vi "Forma Data.vi"(7 "appended array":string[][](array[string]), 8 "error in":errorcluster, 9 "data array":T3 {"data type" items=["Boolean", "SByte", "Byte", "Int16", "UInt16", "Int32", "UInt32", "Int64", "UInt64", "Float", "Double", "String", "DateTime", "ByteString", "Array of Boolean", "Array of SByte", "Array of Byte", "Array of Int16", "Array of UInt16", "Array of Int32", "Array of UInt32", "Array of Int64", "Array of UInt64", "Array of Float", "Array of Double", "Array of String", "Array of DateTime", "Array of ByteString", "Matrix of Boolean", "Matrix of SByte", "Matrix of Byte", "Matrix of Int16", "Matrix of UInt16", "Matrix of Int32", "Matrix of UInt32", "Matrix of Int64", "Matrix of UInt64", "Matrix of Float", "Matrix of Double", "Matrix of String ", "Matrix of DateTime", "Matrix of ByteString"]; "status code" items=["Good"=0, "Good_SubscriptionTransferred"=2949120, "Good_CompletesAsynchronously"=3014656, "Good_Overload"=3080192, "Good_Clamped"=3145728, "Good_LocalOverride"=9830400, "Good_EntryInserted"=10616832, "Good_EntryReplaced"=10682368, "Good_NoData"=10813440, "Good_MoreData"=10878976, "Good_CommunicationEvent"=10944512, "Good_ShutdownEvent"=11010048, "Good_CallAgain"=11075584, "Good_NonCriticalTimeout"=11141120, "Good_ResultsMayBeIncomplete"=12189696, "Good_DataIgnored"=14221312, "Uncertain"=1073741824, "Uncertain_ReferenceOutOfServer"=1080819712, "Uncertain_NoCommunicationLastUsableValue"=1083113472, "Uncertain_LastUsableValue"=1083179008, "Uncertain_SubstituteValue"=1083244544, "Uncertain_InitialValue"=1083310080, "Uncertain_SensorNotAccurate"=1083375616, "Uncertain_EngineeringUnitsExceeded"=1083441152, "Uncertain_SubNormal"=1083506688, "Uncertain_DataSubNormal"=1084489728, "Uncertain_ReferenceNotDeleted"=1086062592, "Uncertain_NotAllNodesAvailable"=1086324736, "Bad"=2147483648, "Bad_UnexpectedError"=2147549184, "Bad_InternalError"=2147614720, "Bad_OutOfMemory"=2147680256, "Bad_ResourceUnavailable"=2147745792, "Bad_CommunicationError"=2147811328, "Bad_EncodingError"=2147876864, "Bad_DecodingError"=2147942400, "Bad_EncodingLimitsExceeded"=2148007936, "Bad_UnknownResponse"=2148073472, "Bad_Timeout"=2148139008, "Bad_ServiceUnsupported"=2148204544, "Bad_Shutdown"=2148270080, "Bad_ServerNotConnected"=2148335616, "Bad_ServerHalted"=2148401152, "Bad_NothingToDo"=2148466688, "Bad_TooManyOperations"=2148532224, "Bad_DataTypeIdUnknown"=2148597760, "Bad_CertificateInvalid"=2148663296, "Bad_SecurityChecksFailed"=2148728832, "Bad_CertificateTimeInvalid"=2148794368, "Bad_CertificateIssuerTimeInvalid"=2148859904, "Bad_CertificateHostNameInvalid"=2148925440, "Bad_CertificateUriInvalid"=2148990976, "Bad_CertificateUseNotAllowed"=2149056512, "Bad_CertificateIssuerUseNotAllowed"=2149122048, "Bad_CertificateUntrusted"=2149187584, "Bad_CertificateRevocationUnknown"=2149253120, "Bad_CertificateIssuerRevocationUnknown"=2149318656, "Bad_CertificateRevoked"=2149384192, "Bad_CertificateIssuerRevoked"=2149449728, "Bad_UserAccessDenied"=2149515264, "Bad_IdentityTokenInvalid"=2149580800, "Bad_IdentityTokenRejected"=2149646336, "Bad_SecureChannelIdInvalid"=2149711872, "Bad_InvalidTimestamp"=2149777408, "Bad_NonceInvalid"=2149842944, "Bad_SessionIdInvalid"=2149908480, "Bad_SessionClosed"=2149974016, "Bad_SessionNotActivated"=2150039552, "Bad_SubscriptionIdInvalid"=2150105088, "Bad_RequestHeaderInvalid"=2150236160, "Bad_TimestampsToReturnInvalid"=2150301696, "Bad_RequestCancelledByClient"=2150367232, "Bad_NoCommunication"=2150694912, "Bad_WaitingForInitialData"=2150760448, "Bad_NodeIdInvalid"=2150825984, "Bad_NodeIdUnknown"=2150891520, "Bad_AttributeIdInvalid"=2150957056, "Bad_IndexRangeInvalid"=2151022592, "Bad_IndexRangeNoData"=2151088128, "Bad_DataEncodingInvalid"=2151153664, "Bad_DataEncodingUnsupported"=2151219200, "Bad_NotReadable"=2151284736, "Bad_NotWritable"=2151350272, "Bad_OutOfRange"=2151415808, "Bad_NotSupported"=2151481344, "Bad_NotFound"=2151546880, "Bad_ObjectDeleted"=2151612416, "Bad_NotImplemented"=2151677952, "Bad_MonitoringModeInvalid"=2151743488, "Bad_MonitoredItemIdInvalid"=2151809024, "Bad_MonitoredItemFilterInvalid"=2151874560, "Bad_MonitoredItemFilterUnsupported"=2151940096, "Bad_FilterNotAllowed"=2152005632, "Bad_StructureMissing"=2152071168, "Bad_EventFilterInvalid"=2152136704, "Bad_ContentFilterInvalid"=2152202240, "Bad_FilterOperandInvalid"=2152267776, "Bad_ContinuationPointInvalid"=2152333312, "Bad_NoContinuationPoints"=2152398848, "Bad_ReferenceTypeIdInvalid"=2152464384, "Bad_BrowseDirectionInvalid"=2152529920, "Bad_NodeNotInView"=2152595456, "Bad_ServerUriInvalid"=2152660992, "Bad_ServerNameMissing"=2152726528, "Bad_DiscoveryUrlMissing"=2152792064, "Bad_SempahoreFileMissing"=2152857600, "Bad_RequestTypeInvalid"=2152923136, "Bad_SecurityModeRejected"=2152988672, "Bad_SecurityPolicyRejected"=2153054208, "Bad_TooManySessions"=2153119744, "Bad_UserSignatureInvalid"=2153185280, "Bad_ApplicationSignatureInvalid"=2153250816, "Bad_NoValidCertificates"=2153316352, "Bad_RequestCancelledByRequest"=2153381888, "Bad_ParentNodeIdInvalid"=2153447424, "Bad_ReferenceNotAllowed"=2153512960, "Bad_NodeIdRejected"=2153578496, "Bad_NodeIdExists"=2153644032, "Bad_NodeClassInvalid"=2153709568, "Bad_BrowseNameInvalid"=2153775104, "Bad_BrowseNameDuplicated"=2153840640, "Bad_NodeAttributesInvalid"=2153906176, "Bad_TypeDefinitionInvalid"=2153971712, "Bad_SourceNodeIdInvalid"=2154037248, "Bad_TargetNodeIdInvalid"=2154102784, "Bad_DuplicateReferenceNotAllowed"=2154168320, "Bad_InvalidSelfReference"=2154233856, "Bad_ReferenceLocalOnly"=2154299392, "Bad_NoDeleteRights"=2154364928, "Bad_ServerIndexInvalid"=2154430464, "Bad_ViewIdUnknown"=2154496000, "Bad_TooManyMatches"=2154627072, "Bad_QueryTooComplex"=2154692608, "Bad_NoMatch"=2154758144, "Bad_MaxAgeInvalid"=2154823680, "Bad_HistoryOperationInvalid"=2154889216, "Bad_HistoryOperationUnsupported"=2154954752, "Bad_WriteNotSupported"=2155020288, "Bad_TypeMismatch"=2155085824, "Bad_MethodInvalid"=2155151360, "Bad_ArgumentsMissing"=2155216896, "Bad_TooManySubscriptions"=2155282432, "Bad_TooManyPublishRequests"=2155347968, "Bad_NoSubscription"=2155413504, "Bad_SequenceNumberUnknown"=2155479040, "Bad_MessageNotAvailable"=2155544576, "Bad_InsufficientClientProfile"=2155610112, "Bad_TcpServerTooBusy"=2155675648, "Bad_TcpMessageTypeInvalid"=2155741184, "Bad_TcpSecureChannelUnknown"=2155806720, "Bad_TcpMessageTooLarge"=2155872256, "Bad_TcpNotEnoughResources"=2155937792, "Bad_TcpInternalError"=2156003328, "Bad_TcpEndpointUrlInvalid"=2156068864, "Bad_RequestInterrupted"=2156134400, "Bad_RequestTimeout"=2156199936, "Bad_SecureChannelClosed"=2156265472, "Bad_SecureChannelTokenUnknown"=2156331008, "Bad_SequenceNumberInvalid"=2156396544, "Bad_ConfigurationError"=2156462080, "Bad_NotConnected"=2156527616, "Bad_DeviceFailure"=2156593152, "Bad_SensorFailure"=2156658688, "Bad_OutOfService"=2156724224, "Bad_DeadbandFilterInvalid"=2156789760, "Bad_RefreshInProgress"=2157379584, "Bad_ConditionAlreadyDisabled"=2157445120, "Bad_ConditionDisabled"=2157510656, "Bad_EventIdUnknown"=2157576192, "Bad_NoData"=2157641728, "Bad_DataLost"=2157772800, "Bad_DataUnavailable"=2157838336, "Bad_EntryExists"=2157903872, "Bad_NoEntryExists"=2157969408, "Bad_TimestampNotSupported"=2158034944, "Bad_InvalidArgument"=2158690304, "Bad_ConnectionRejected"=2158755840, "Bad_Disconnect"=2158821376, "Bad_ConnectionClosed"=2158886912, "Bad_InvalidState"=2158952448, "Bad_EndOfStream"=2159017984, "Bad_NoDataAvailable"=2159083520, "Bad_WaitingForResponse"=2159149056, "Bad_OperationAbandoned"=2159214592, "Bad_ExpectedStreamToBlock"=2159280128, "Bad_WouldBlock"=2159345664, "Bad_SyntaxError"=2159411200, "Bad_MaxConnectionsReached"=2159476736, "Bad_RequestTooLarge"=2159542272, "Bad_ResponseTooLarge"=2159607808, "Bad_EventNotAcknowledgeable"=2159738880, "Bad_InvalidTimestampArgument"=2159869952, "Bad_ProtocolVersionUnsupported"=2159935488, "Bad_StateNotActive"=2160001024, "Bad_FilterOperatorInvalid"=2160132096, "Bad_FilterOperatorUnsupported"=2160197632, "Bad_FilterOperandCountMismatch"=2160263168, "Bad_FilterElementInvalid"=2160328704, "Bad_FilterLiteralInvalid"=2160394240, "Bad_IdentityChangeNotSupported"=2160459776, "Bad_NotTypeDefinition"=2160590848, "Bad_ViewTimestampInvalid"=2160656384, "Bad_ViewParameterMismatch"=2160721920, "Bad_ViewVersionInvalid"=2160787456, "Bad_ConditionAlreadyEnabled"=2160852992, "Bad_DialogNotActive"=2160918528, "Bad_DialogResponseInvalid"=2160984064, "Bad_ConditionBranchAlreadyAcked"=2161049600, "Bad_ConditionBranchAlreadyConfirmed"=2161115136, "Bad_ConditionAlreadyShelved"=2161180672, "Bad_ConditionNotShelved"=2161246208, "Bad_ShelvingTimeOutOfRange"=2161311744, "Bad_AggregateListMismatch"=2161377280, "Bad_AggregateNotSupported"=2161442816, "Bad_AggregateInvalidInputs"=2161508352, "Bad_BoundNotFound"=2161573888, "Bad_BoundNotSupported"=2161639424, "Bad_AggregateConfigurationRejected"=2161770496, "Bad_TooManyMonitoredItems"=2161836032]}, 10 "type":enum16{"Insert", "Replace", "Append"}(ring), 11 "Multicolumn Listbox":refnum<vi>) -> (0 "error out":errorcluster, 1 "Alarm Summary Data":string[][](array[string]), 2 "Alarm Summary Headers":string[](array[string]), 3 "dup Multicolumn Listbox":refnum<vi>)   [LabVIEW 2019]
uses:
  Alarm Description Item.ctl
  Control 1.ctl
  <vilib>/OPCUA/controls/Subscription Data Change.ctl
  <vilib>/OPCUA/controls/NodeId.ctl
  <vilib>/OPCUA/controls/Data Type.ctl
  <vilib>/OPCUA/controls/OPC UA StatusCode.ctl
panel:
  out "data type":T1=1 items=["Boolean", "SByte", "Byte", "Int16", "UInt16", "Int32", "UInt32", "Int64", "UInt64", "Float", "Double", "String", "DateTime", "ByteString", "Array of Boolean", "Array of SByte", "Array of Byte", "Array of Int16", "Array of UInt16", "Array of Int32", "Array of UInt32", "Array of Int64", "Array of UInt64", "Array of Float", "Array of Double", "Array of String", "Array of DateTime", "Array of ByteString", "Matrix of Boolean", "Matrix of SByte", "Matrix of Byte", "Matrix of Int16", "Matrix of UInt16", "Matrix of Int32", "Matrix of UInt32", "Matrix of Int64", "Matrix of UInt64", "Matrix of Float", "Matrix of Double", "Matrix of String ", "Matrix of DateTime", "Matrix of ByteString"]
  out "Status Code":T2 items=["Good"=0, "Good_SubscriptionTransferred"=2949120, "Good_CompletesAsynchronously"=3014656, "Good_Overload"=3080192, "Good_Clamped"=3145728, "Good_LocalOverride"=9830400, "Good_EntryInserted"=10616832, "Good_EntryReplaced"=10682368, "Good_NoData"=10813440, "Good_MoreData"=10878976, "Good_CommunicationEvent"=10944512, "Good_ShutdownEvent"=11010048, "Good_CallAgain"=11075584, "Good_NonCriticalTimeout"=11141120, "Good_ResultsMayBeIncomplete"=12189696, "Good_DataIgnored"=14221312, "Uncertain"=1073741824, "Uncertain_ReferenceOutOfServer"=1080819712, "Uncertain_NoCommunicationLastUsableValue"=1083113472, "Uncertain_LastUsableValue"=1083179008, "Uncertain_SubstituteValue"=1083244544, "Uncertain_InitialValue"=1083310080, "Uncertain_SensorNotAccurate"=1083375616, "Uncertain_EngineeringUnitsExceeded"=1083441152, "Uncertain_SubNormal"=1083506688, "Uncertain_DataSubNormal"=1084489728, "Uncertain_ReferenceNotDeleted"=1086062592, "Uncertain_NotAllNodesAvailable"=1086324736, "Bad"=2147483648, "Bad_UnexpectedError"=2147549184, "Bad_InternalError"=2147614720, "Bad_OutOfMemory"=2147680256, "Bad_ResourceUnavailable"=2147745792, "Bad_CommunicationError"=2147811328, "Bad_EncodingError"=2147876864, "Bad_DecodingError"=2147942400, "Bad_EncodingLimitsExceeded"=2148007936, "Bad_UnknownResponse"=2148073472, "Bad_Timeout"=2148139008, "Bad_ServiceUnsupported"=2148204544, "Bad_Shutdown"=2148270080, "Bad_ServerNotConnected"=2148335616, "Bad_ServerHalted"=2148401152, "Bad_NothingToDo"=2148466688, "Bad_TooManyOperations"=2148532224, "Bad_DataTypeIdUnknown"=2148597760, "Bad_CertificateInvalid"=2148663296, "Bad_SecurityChecksFailed"=2148728832, "Bad_CertificateTimeInvalid"=2148794368, "Bad_CertificateIssuerTimeInvalid"=2148859904, "Bad_CertificateHostNameInvalid"=2148925440, "Bad_CertificateUriInvalid"=2148990976, "Bad_CertificateUseNotAllowed"=2149056512, "Bad_CertificateIssuerUseNotAllowed"=2149122048, "Bad_CertificateUntrusted"=2149187584, "Bad_CertificateRevocationUnknown"=2149253120, "Bad_CertificateIssuerRevocationUnknown"=2149318656, "Bad_CertificateRevoked"=2149384192, "Bad_CertificateIssuerRevoked"=2149449728, "Bad_UserAccessDenied"=2149515264, "Bad_IdentityTokenInvalid"=2149580800, "Bad_IdentityTokenRejected"=2149646336, "Bad_SecureChannelIdInvalid"=2149711872, "Bad_InvalidTimestamp"=2149777408, "Bad_NonceInvalid"=2149842944, "Bad_SessionIdInvalid"=2149908480, "Bad_SessionClosed"=2149974016, "Bad_SessionNotActivated"=2150039552, "Bad_SubscriptionIdInvalid"=2150105088, "Bad_RequestHeaderInvalid"=2150236160, "Bad_TimestampsToReturnInvalid"=2150301696, "Bad_RequestCancelledByClient"=2150367232, "Bad_NoCommunication"=2150694912, "Bad_WaitingForInitialData"=2150760448, "Bad_NodeIdInvalid"=2150825984, "Bad_NodeIdUnknown"=2150891520, "Bad_AttributeIdInvalid"=2150957056, "Bad_IndexRangeInvalid"=2151022592, "Bad_IndexRangeNoData"=2151088128, "Bad_DataEncodingInvalid"=2151153664, "Bad_DataEncodingUnsupported"=2151219200, "Bad_NotReadable"=2151284736, "Bad_NotWritable"=2151350272, "Bad_OutOfRange"=2151415808, "Bad_NotSupported"=2151481344, "Bad_NotFound"=2151546880, "Bad_ObjectDeleted"=2151612416, "Bad_NotImplemented"=2151677952, "Bad_MonitoringModeInvalid"=2151743488, "Bad_MonitoredItemIdInvalid"=2151809024, "Bad_MonitoredItemFilterInvalid"=2151874560, "Bad_MonitoredItemFilterUnsupported"=2151940096, "Bad_FilterNotAllowed"=2152005632, "Bad_StructureMissing"=2152071168, "Bad_EventFilterInvalid"=2152136704, "Bad_ContentFilterInvalid"=2152202240, "Bad_FilterOperandInvalid"=2152267776, "Bad_ContinuationPointInvalid"=2152333312, "Bad_NoContinuationPoints"=2152398848, "Bad_ReferenceTypeIdInvalid"=2152464384, "Bad_BrowseDirectionInvalid"=2152529920, "Bad_NodeNotInView"=2152595456, "Bad_ServerUriInvalid"=2152660992, "Bad_ServerNameMissing"=2152726528, "Bad_DiscoveryUrlMissing"=2152792064, "Bad_SempahoreFileMissing"=2152857600, "Bad_RequestTypeInvalid"=2152923136, "Bad_SecurityModeRejected"=2152988672, "Bad_SecurityPolicyRejected"=2153054208, "Bad_TooManySessions"=2153119744, "Bad_UserSignatureInvalid"=2153185280, "Bad_ApplicationSignatureInvalid"=2153250816, "Bad_NoValidCertificates"=2153316352, "Bad_RequestCancelledByRequest"=2153381888, "Bad_ParentNodeIdInvalid"=2153447424, "Bad_ReferenceNotAllowed"=2153512960, "Bad_NodeIdRejected"=2153578496, "Bad_NodeIdExists"=2153644032, "Bad_NodeClassInvalid"=2153709568, "Bad_BrowseNameInvalid"=2153775104, "Bad_BrowseNameDuplicated"=2153840640, "Bad_NodeAttributesInvalid"=2153906176, "Bad_TypeDefinitionInvalid"=2153971712, "Bad_SourceNodeIdInvalid"=2154037248, "Bad_TargetNodeIdInvalid"=2154102784, "Bad_DuplicateReferenceNotAllowed"=2154168320, "Bad_InvalidSelfReference"=2154233856, "Bad_ReferenceLocalOnly"=2154299392, "Bad_NoDeleteRights"=2154364928, "Bad_ServerIndexInvalid"=2154430464, "Bad_ViewIdUnknown"=2154496000, "Bad_TooManyMatches"=2154627072, "Bad_QueryTooComplex"=2154692608, "Bad_NoMatch"=2154758144, "Bad_MaxAgeInvalid"=2154823680, "Bad_HistoryOperationInvalid"=2154889216, "Bad_HistoryOperationUnsupported"=2154954752, "Bad_WriteNotSupported"=2155020288, "Bad_TypeMismatch"=2155085824, "Bad_MethodInvalid"=2155151360, "Bad_ArgumentsMissing"=2155216896, "Bad_TooManySubscriptions"=2155282432, "Bad_TooManyPublishRequests"=2155347968, "Bad_NoSubscription"=2155413504, "Bad_SequenceNumberUnknown"=2155479040, "Bad_MessageNotAvailable"=2155544576, "Bad_InsufficientClientProfile"=2155610112, "Bad_TcpServerTooBusy"=2155675648, "Bad_TcpMessageTypeInvalid"=2155741184, "Bad_TcpSecureChannelUnknown"=2155806720, "Bad_TcpMessageTooLarge"=2155872256, "Bad_TcpNotEnoughResources"=2155937792, "Bad_TcpInternalError"=2156003328, "Bad_TcpEndpointUrlInvalid"=2156068864, "Bad_RequestInterrupted"=2156134400, "Bad_RequestTimeout"=2156199936, "Bad_SecureChannelClosed"=2156265472, "Bad_SecureChannelTokenUnknown"=2156331008, "Bad_SequenceNumberInvalid"=2156396544, "Bad_ConfigurationError"=2156462080, "Bad_NotConnected"=2156527616, "Bad_DeviceFailure"=2156593152, "Bad_SensorFailure"=2156658688, "Bad_OutOfService"=2156724224, "Bad_DeadbandFilterInvalid"=2156789760, "Bad_RefreshInProgress"=2157379584, "Bad_ConditionAlreadyDisabled"=2157445120, "Bad_ConditionDisabled"=2157510656, "Bad_EventIdUnknown"=2157576192, "Bad_NoData"=2157641728, "Bad_DataLost"=2157772800, "Bad_DataUnavailable"=2157838336, "Bad_EntryExists"=2157903872, "Bad_NoEntryExists"=2157969408, "Bad_TimestampNotSupported"=2158034944, "Bad_InvalidArgument"=2158690304, "Bad_ConnectionRejected"=2158755840, "Bad_Disconnect"=2158821376, "Bad_ConnectionClosed"=2158886912, "Bad_InvalidState"=2158952448, "Bad_EndOfStream"=2159017984, "Bad_NoDataAvailable"=2159083520, "Bad_WaitingForResponse"=2159149056, "Bad_OperationAbandoned"=2159214592, "Bad_ExpectedStreamToBlock"=2159280128, "Bad_WouldBlock"=2159345664, "Bad_SyntaxError"=2159411200, "Bad_MaxConnectionsReached"=2159476736, "Bad_RequestTooLarge"=2159542272, "Bad_ResponseTooLarge"=2159607808, "Bad_EventNotAcknowledgeable"=2159738880, "Bad_InvalidTimestampArgument"=2159869952, "Bad_ProtocolVersionUnsupported"=2159935488, "Bad_StateNotActive"=2160001024, "Bad_FilterOperatorInvalid"=2160132096, "Bad_FilterOperatorUnsupported"=2160197632, "Bad_FilterOperandCountMismatch"=2160263168, "Bad_FilterElementInvalid"=2160328704, "Bad_FilterLiteralInvalid"=2160394240, "Bad_IdentityChangeNotSupported"=2160459776, "Bad_NotTypeDefinition"=2160590848, "Bad_ViewTimestampInvalid"=2160656384, "Bad_ViewParameterMismatch"=2160721920, "Bad_ViewVersionInvalid"=2160787456, "Bad_ConditionAlreadyEnabled"=2160852992, "Bad_DialogNotActive"=2160918528, "Bad_DialogResponseInvalid"=2160984064, "Bad_ConditionBranchAlreadyAcked"=2161049600, "Bad_ConditionBranchAlreadyConfirmed"=2161115136, "Bad_ConditionAlreadyShelved"=2161180672, "Bad_ConditionNotShelved"=2161246208, "Bad_ShelvingTimeOutOfRange"=2161311744, "Bad_AggregateListMismatch"=2161377280, "Bad_AggregateNotSupported"=2161442816, "Bad_AggregateInvalidInputs"=2161508352, "Bad_BoundNotFound"=2161573888, "Bad_BoundNotSupported"=2161639424, "Bad_AggregateConfigurationRejected"=2161770496, "Bad_TooManyMonitoredItems"=2161836032]
  in  "alarm display format":T6[](array[typedef])=[enum."Type", enum."Name", enum."Value", enum."time", enum."status code", enum."data type", enum."node ID", enum."Color"]
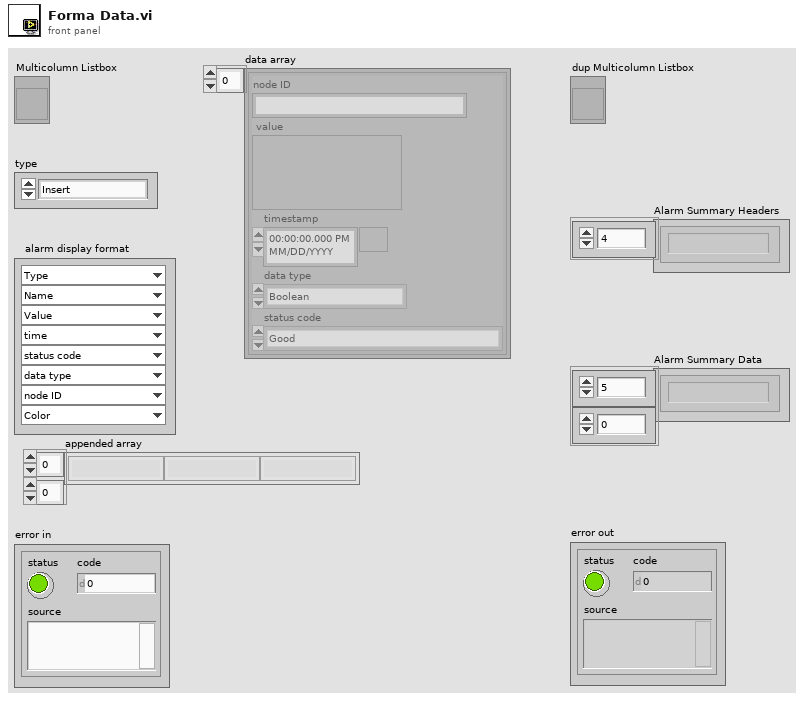
[diagram p1: front panel]
types:
  T1 = typedef "Data Type.ctl" = u16
  T2 = typedef "OPC UA StatusCode.ctl" = u32
  T3 = typedef "Control 1.ctl" = T4[]
  T4 = typedef "Subscription Data Change.ctl" = cluster{"node ID":T5, " value":variant, "timestamp":timestamp, "data type":T1, "status code":T2}
  T5 = typedef "NodeId.ctl" = string
  T6 = typedef "Alarm Description Item.ctl" = enum16{"Type", "Name", "node ID", "Value", "time", "data type", "status code", "Color"}
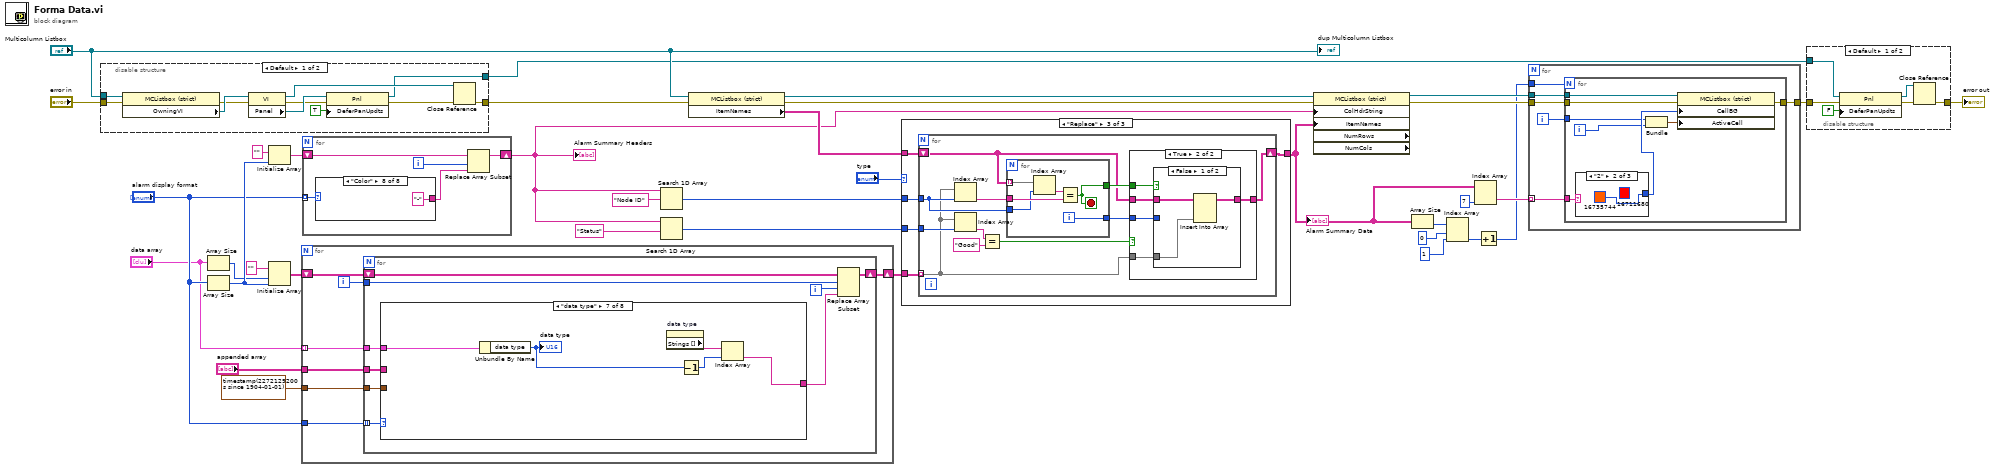
[diagram p0: block diagram]
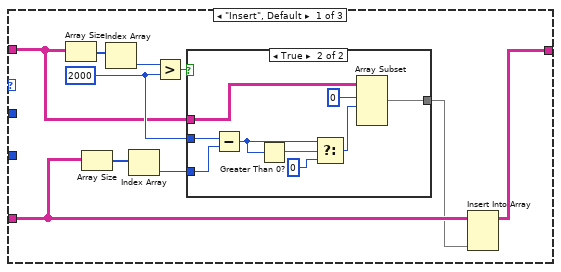
[diagram p4: hidden frame]
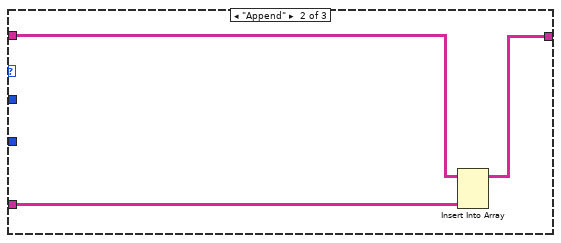
[diagram p6: hidden frame]
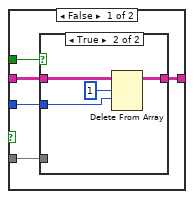
[diagram p7: hidden frame]
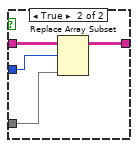
[diagram p9: hidden frame]
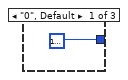
[diagram p10: hidden frame]
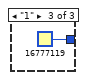
[diagram p11: hidden frame]
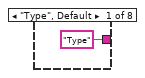
[diagram p12: hidden frame]
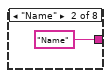
[diagram p13: hidden frame]
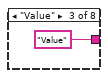
[diagram p14: hidden frame]
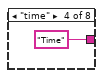
[diagram p15: hidden frame]
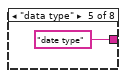
[diagram p16: hidden frame]
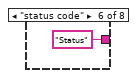
[diagram p17: hidden frame]
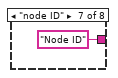
[diagram p18: hidden frame]
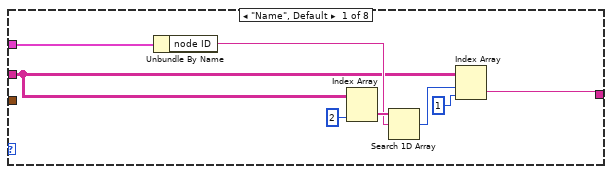
[diagram p19: hidden frame]
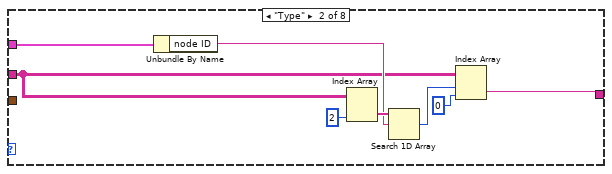
[diagram p20: hidden frame]
diagram:
  n1 = disable-structure shown="Default" {
    disable-tunnel: "error in" -> [w40 w48]
    disable-tunnel: "Multicolumn Listbox" -> [w39 _]
    disable-tunnel: [w38 w48] -> w14
    disable-tunnel: [w37 _] -> w11
    frame condition #0 (active) {
      n2 = property class="MCListbox (strict)"(reference=w39, error in=w40) -> (error out=w46:errorcluster, "OwningVI"=w47:refnum<vi>)  [unwired: 1 out]
      n3 = property class="VI"(reference=w47, error in=w46) -> (reference out=w42:refnum<vi>, error out=w44:errorcluster, "Panel"=w45:refnum<vi>)
      n4 = property class="Pnl"(reference=w45, error in=w44, "DeferPanUpdts"=TRUE ("Defer Panel Updates")) -> (reference out=w37:refnum<vi>, error out=w41:errorcluster)
      n5 = Close Reference(reference=w42, error in (no error)=w41) -> (error out=w38:errorcluster)
    }
    frame condition #1 {
    }
  }
  n6 = Array Size(array="data array") -> (size(s)=w31:i32)
  n7 = Array Size(array="alarm display format") -> (size(s)=w35:i32)
  n8 = Initialize Array("" ("element"), w35) -> (w36:string[])
  n9 = Initialize Array("" ("alarm URL"), w31, w35) -> (w33:string[][])
  n10 = for {
    tunnel: "data array" -> [w50] mode=indexing
    tunnel: "alarm display format" -> [w55]
    shift-right: [w53] -> w21
    shift-left: w33 -> [w54]
    tunnel: timestamp(2272129200 s since 1904-01-01) ("ack time") -> [w51]
    tunnel: "appended array" -> [w49]
    i -> [w52]
    n11 = for {
      tunnel: w55 -> [w64] mode=indexing
      tunnel: w50 -> [w57]
      tunnel: w52 -> [w61]
      shift-right: [w62] -> w53
      shift-left: w54 -> [w63]
      tunnel: w51 -> [w58]
      tunnel: w49 -> [w56]
      i -> [w60]
      n12 = case shown="\"data type\"" w64 {
        tunnel: w57 -> [w72 w80 w92 w100 w107 w112 w121 w125]
        tunnel: [w66 w73 w81 w99 w102 w111 w119 w122] -> w59
        tunnel: w58 -> [_ _ _ _ _ w109 _ _]
        tunnel: w56 -> [w65 w74 w86 _ _ _ _ _]
        frame "Name", Default {
          n13 = Unbundle By Name(w72) -> ("node ID"=w69:T5)
          n14 = Index Array(array=w65, index (col)=2 ("disabled index (col)")) -> (element=w70:string[])  [unwired: 1 in]
          n15 = Search 1D Array(1D array=w70, element=w69) -> (index of element=w67:i32)  [unwired: 1 in]
          n16 = Index Array(array=w65, index (row)=w67, index (col)=1 ("disabled index (col)")) -> (element=w66:string)
        }
        frame "Type" {
          n17 = Unbundle By Name(w80) -> ("node ID"=w77:T5)
          n18 = Index Array(array=w74, index (col)=2 ("disabled index (col)")) -> (element=w78:string[])  [unwired: 1 in]
          n19 = Search 1D Array(1D array=w78, element=w77) -> (index of element=w75:i32)  [unwired: 1 in]
          n20 = Index Array(array=w74, index (row)=w75, index (col)=0 ("disabled index (col)")) -> (element=w73:string)
        }
        frame "Color" {
          n21 = Unbundle By Name(w92) -> ("value"=w83:variant, "node ID"=w89:T5)
          n22 = Index Array(array=w86, index (col)=2 ("disabled index (col)")) -> (element=w90:string[])  [unwired: 1 in]
          n23 = Search 1D Array(1D array=w90, element=w89) -> (index of element=w87:i32)  [unwired: 1 in]
          n24 = Variant To Data(type=FALSE, Variant=w83) -> (data=w82:bool)  [unwired: 1 in, 1 out]
          n25 = Index Array(array=w86, index (row)=w87, index (col)=0 ("disabled index (col)")) -> (element=w85:string)
          n26 = case shown="True" w82 {
            tunnel: w85 -> [_ w95]
            tunnel: ["0" w94] -> w81
            frame False {
            }
            frame True {
              n27 = case shown="\"Warning\"" w95 {
                tunnel: ["0" "2" "1"] -> w94
                frame "False", Default {
                }
                frame "Alarm" {
                }
                frame "Warning" {
                }
              }
            }
          }
        }
        frame "node ID" {
          n28 = Unbundle By Name(w100) -> ("node ID"=w99:T5)
        }
        frame "Value" {
          n29 = Unbundle By Name(w107) -> ("value"=w105:variant)
          n30 = Variant To Data(type=FALSE, Variant=w105) -> (data=w101:bool)  [unwired: 1 in, 1 out]
          n31 = Select(t="True" ("alarm URL"), s=w101, f="False") -> (s? t:f=w102:string)
        }
        frame "time" {
          n32 = Unbundle By Name(w112) -> ("timestamp"=w108:timestamp)
          n33 = Less?(x=w108, y=w109) -> (x < y?=w110:bool)
          n34 = case shown="False" w110 {
            tunnel: w108 -> [w115 _]
            tunnel: [w113 "" ("date/time string")] -> w111
            frame False {
              n35 = Format Date/Time String(time format string (%c)="%m/%d/%Y %H:%M:%S", seconds (now)=w115) -> (date/time string=w113:string)  [unwired: 1 in]
            }
            frame True {
            }
          }
        }
        frame "data type" {
          n36 = Unbundle By Name(w121) -> ("data type"=w117:T1)
          "data type" <- w117
          n37 = property on="data type" class="Ring (strict)"() -> ("Strings []"=w120:string[])  [unwired: 2 in, 2 out]
          n38 = Decrement(x=w117) -> (x-1=w118:T1)
          n39 = Index Array(array=w120, index=w118) -> (element=w119:string)
        }
        frame "status code" {
          n40 = Unbundle By Name(w125) -> ("status code"=w123:T2)
          "Status Code" <- w123
          n41 = property on="Status Code" class="Ring (strict)"() -> ("Strings []"=w124:string[])  [unwired: 2 in, 2 out]
          n42 = Index Array(array=w124, index=w123) -> (element=w122:string)
        }
      }
      n43 = Replace Array Subset(array=w63, new element=w59, index (row)=w61, index (col)=w60) -> (w62:string[][])
    }
  }
  n44 = for {
    tunnel: "alarm display format" -> [w130] mode=indexing
    shift-right: [w128] -> w20
    shift-left: w36 -> [w129]
    i -> [w127]
    n45 = case shown="\"Color\"" w130 {
      tunnel: ["Type" ("element") "Name" ("element") "Value" ("element") "Time" ("element") "date type" ("element") "Status" ("element") "Node ID" ("element") "-" ("element")] -> w126
      frame "Type", Default {
      }
      frame "Name" {
      }
      frame "Value" {
      }
      frame "time" {
      }
      frame "data type" {
      }
      frame "status code" {
      }
      frame "node ID" {
      }
      frame "Color" {
      }
    }
    n46 = Replace Array Subset(array=w129, new element=w126, index=w127) -> (w128:string[])
  }
  "Alarm Summary Headers" <- w20
  n47 = Search 1D Array(1D array=w20, element="Node ID") -> (index of element=w18:i32)  [unwired: 1 in]
  n48 = Search 1D Array(1D array=w20, element="Status") -> (index of element=w17:i32)  [unwired: 1 in]
  n49 = property class="MCListbox (strict)"(reference="Multicolumn Listbox", error in=w14) -> (reference out=w24:refnum<vi>, error out=w25:errorcluster, "ItemNames"=w22:string[][])
  n50 = case shown="\"Replace\"" "type" {
    tunnel: w22 -> [w139 w159 w165]
    tunnel: w21 -> [w145 w160 w166]
    tunnel: [w146 w161 w162] -> w4
    tunnel: w18 -> [_ _ w164]
    tunnel: w17 -> [_ _ w163]
    frame "Insert", Default {
      w141 = 2000 ("y")
      n51 = Array Size(array=w139) -> (size(s)=w148:i32[])
      n52 = Array Size(array=w145) -> (size(s)=w144:i32[])
      n53 = Index Array(array=w148) -> (element=w142:i32)  [unwired: 1 in]
      n54 = Index Array(array=w144) -> (element=w143:i32)  [unwired: 1 in]
      n55 = Greater?(x=w142, y=w141) -> (0:w147:bool)
      n56 = case shown="True" w147 {
        tunnel: w139 -> [w149 w158]
        tunnel: w143 -> [_ w156]
        tunnel: w141 -> [_ w157]
        tunnel: [w149 w150] -> w140
        frame False {
        }
        frame True {
          n57 = Subtract(x=w157, y=w156) -> (x-y=w154:i32)
          n58 = Greater Than 0?(x=w154) -> (x > 0?=w155:bool)
          n59 = Select(t=w154, s=w155, f=0) -> (s? t:f=w151:i32)
          n60 = Array Subset(array=w158, index (row)=0, length (row)=w151) -> (w150:string[][])  [unwired: 2 in]
        }
      }
      n61 = Insert Into Array(array=w145, new element=w140) -> (w146:string[][])  [unwired: 2 in]
    }
    frame "Append" {
      n62 = Insert Into Array(array=w159, new element=w160) -> (w161:string[][])  [unwired: 2 in]
    }
    frame "Replace" {
      n63 = for {
        tunnel: w166 -> [w168] mode=indexing
        tunnel: w164 -> [w169]
        tunnel: w163 -> [w170]
        shift-right: [w167] -> w162
        shift-left: w165 -> [w171]
        n64 = Index Array(array=w168, index=w169) -> (element=w177:string)
        n65 = Index Array(array=w168, index=w170) -> (element=w175:string)
        n66 = Equal?(x=w175, y="Good" ("f")) -> (x = y?=w173:bool)
        n67 = for {
          tunnel: [w205] -> w174
          tunnel: [w204] -> w172
          tunnel: w171 -> [w203] mode=indexing
          tunnel: w177 -> [w201]
          tunnel: w169 -> [w200]
          i -> [w204]
          stop <- w205 stop-if-true
          n68 = Index Array(array=w203, index=w200) -> (element=w202:string)
          n69 = Equal?(x=w202, y=w201) -> (x = y?=w205:bool)
        }
        n70 = case shown="True" w173 {
          tunnel: w174 -> [w182 w192]
          tunnel: w172 -> [w178 w191]
          tunnel: w171 -> [w180 w190]
          tunnel: w168 -> [w181 w189]
          tunnel: [w179 w188] -> w167
          frame False {
            n71 = case shown="True" w182 {
              tunnel: w181 -> [_ _]
              tunnel: w180 -> [w183 w187]
              tunnel: [w183 w185] -> w179
              tunnel: w178 -> [_ w184]
              frame False {
              }
              frame True {
                n72 = Delete From Array(array=w187, length=1, index (row)=w184) -> (array with subset deleted=w185:string[][])  [unwired: 1 in, 1 out]
              }
            }
          }
          frame True {
            n73 = case shown="False" w192 {
              tunnel: w191 -> [_ w198]
              tunnel: w190 -> [w195 w199]
              tunnel: w189 -> [w194 w197]
              tunnel: [w193 w196] -> w188
              frame False {
                n74 = Insert Into Array(array=w195, new element=w194) -> (w193:string[][])  [unwired: 2 in]
              }
              frame True {
                n75 = Replace Array Subset(array=w199, new element=w197, index (row)=w198) -> (w196:string[][])  [unwired: 1 in]
              }
            }
          }
        }
      }
    }
  }
  "Alarm Summary Data" <- w4
  n76 = property class="MCListbox (strict)" props=["ColHdrString", "ItemNames", "NumRows", "NumCols"](reference=w24, error in=w25, "ColHdrString"=w20, "ItemNames"=w4) -> (reference out=w29:refnum<vi>, error out=w28:errorcluster)  [unwired: 2 out]
  n77 = Array Size(array=w4) -> (size(s)=w7:i32[])
  n78 = Index Array(array=w7, index #1=0 ("index"), index #2=1 ("index")) -> (element #2=w2:i32)  [unwired: 1 out]
  n79 = Index Array(array=w4, index (col)=7 ("disabled index (col)")) -> (element=w3:string[])  [unwired: 1 in]
  n80 = Increment(x=w2) -> (x+1=w1:i32)
  n81 = for {
    tunnel: [w211] -> w13
    tunnel: w1 -> [w210]
    tunnel: w29 -> [w209]
    tunnel: w28 -> [w208]
    tunnel: w3 -> [w207] mode=indexing
    i -> [w206]
    n82 = for {
      N: w210 -> [_]
      tunnel: w206 -> [w213]
      tunnel: [w219] -> w211
      tunnel: w209 -> [w218]
      tunnel: w208 -> [w217]
      tunnel: w207 -> [w215]
      i -> [w212]
      n83 = case shown="\"2\"" w215 {
        tunnel: [u32 16777226 ("Default BG Color") u32 16735744 u32 16777119] -> w214
        frame "0", Default {
        }
        frame "2" {
          (unwired) u32 16711680
        }
        frame "1" {
        }
      }
      n84 = Bundle(w213, w212) -> (w216:cluster{i32, i32})  [unwired: 1 in]
      n85 = property class="MCListbox (strict)"(reference=w218, error in=w217, "CellBG"=w214, "ActiveCell"=w216) -> (error out=w219:errorcluster)  [unwired: 1 out]
    }
  }
  n86 = disable-structure shown="Default" {
    disable-tunnel: w13 -> [w225 w229]
    disable-tunnel: [w224 w229] -> w12
    disable-tunnel: w11 -> [w223 _]
    frame condition #0 (active) {
      n87 = property class="Pnl"(reference=w223, error in=w225, "DeferPanUpdts"=FALSE ("Defer Panel Updates")) -> (reference out=w226:refnum<vi>, error out=w227:errorcluster)
      n88 = Close Reference(reference=w226, error in (no error)=w227) -> (error out=w224:errorcluster)
    }
    frame condition #1 {
    }
  }
  "error out" <- w12
  "dup Multicolumn Listbox" <- "Multicolumn Listbox"
